vi "DB - Replace String SQL.vi"(1 "DB.Schema.Table":T1[](array[typedef]), 2 "String In":string) -> (0 "String Out":string)   [LabVIEW 2020]
uses:
  Control/DB Schema Table DS.ctl
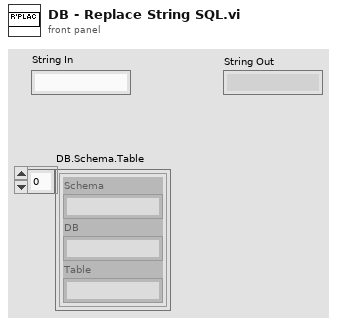
[diagram p1: front panel]
types:
  T1 = typedef "DB Schema Table DS.ctl" = cluster{"Schema":string, "DB":string, "Table":string}
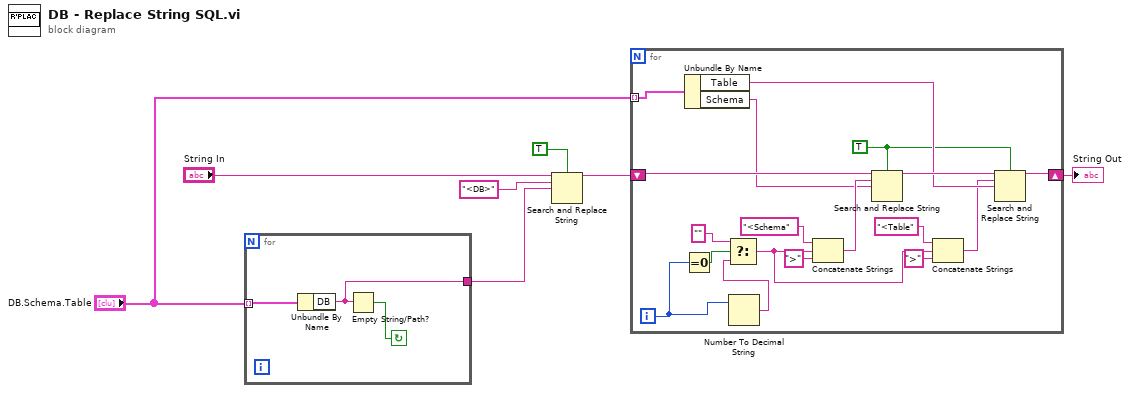
[diagram p0: block diagram]
diagram:
  n1 = for {
    tunnel: "DB.Schema.Table" -> [w10] mode=indexing
    tunnel: [w8] -> w5
    stop <- w9 continue-if-true
    n2 = Unbundle By Name(w10) -> ("DB"=w8:string)
    n3 = Empty String/Path?(string/path=w8) -> (empty?=w9:bool)
  }
  n4 = Search and Replace String(case sensitive?=TRUE ("ignore case? (F)"), input string="String In", search string="<DB>", replace string=w5) -> (result string=w3:string)  [unwired: 4 in, 3 out]
  n5 = for {
    tunnel: "DB.Schema.Table" -> [w28] mode=indexing
    shift-right: [w22] -> w1
    shift-left: w3 -> [w24]
    i -> [w25]
    w12 = TRUE ("ignore case? (F)")
    n6 = Equal To 0?(x=w25) -> (x = 0?=w27:bool)
    n7 = Unbundle By Name(w28) -> ("Table"=w13:string, "Schema"=w14:string)
    n8 = Number To Decimal String(number=w25) -> (decimal integer string=w21:string)  [unwired: 1 in]
    n9 = Select(t="", s=w27, f=w21) -> (s? t:f=w16:string)
    n10 = Concatenate Strings("<Schema" ("string"), w16, ">" ("string")) -> (w15:string)
    n11 = Search and Replace String(case sensitive?=w12, input string=w24, search string=w15, replace string=w14) -> (result string=w23:string)  [unwired: 4 in, 3 out]
    n12 = Concatenate Strings("<Table" ("string"), w16, ">" ("string")) -> (w11:string)
    n13 = Search and Replace String(case sensitive?=w12, input string=w23, search string=w11, replace string=w13) -> (result string=w22:string)  [unwired: 4 in, 3 out]
  }
  "String Out" <- w1
